vi "XSubMenu-Facade.vi"(0 "Data In":T4, 2 "Display State In":T2={"Items"=[{"Tag"="1", "Name"="1", "Symbol"=0, "Checked"=FALSE, "ParentTag"="t"}], "CellHeight"=0}, 3 "Container State":T3) -> (6 "Data Out":T4, 7 "Display State Out":T2={"Items"=[{"Tag"="1", "Name"="1", "Symbol"=0, "Checked"=FALSE, "ParentTag"="t"}], "CellHeight"=0}, 8 "Action":T1)   [LabVIEW 2020, in "XSubMenu.xctl"]
uses:
  XSubMenu.xctl
  XSubMenu-Data.ctl
  <vilib>/_xctls/Container State.ctl
  XSubMenu-State.ctl
  <vilib>/_xctls/Action.ctl
  <vilib>/_xctls/XControlSupport.lvlib
panel:
  in  "SubMenu":i32(listbox)
  in  "black-ListBg":bool
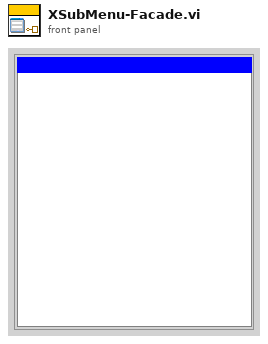
[diagram p1: front panel]
types:
  T1 = typedef "XControlSupport.lvlib/Action.ctl" = cluster{"Data Changed?":bool, "State Changed?":bool, "Action Name":string}
  T2 = typedef "XSubMenu.xctl/XSubMenu-State.ctl" = cluster{"Items":cluster{"Tag":string, "Name":string, "Symbol":i32, "Checked":bool, "ParentTag":string}[], "CellHeight":i32}
  T3 = typedef "XControlSupport.lvlib/Container State.ctl" = cluster{"Indicator?":bool, "Run Mode?":bool, " Refnum":refnum<vi>}
  T4 = typedef "XSubMenu.xctl/XSubMenu-Data.ctl" = i32
  T5 = cluster{"Tag":string, "Name":string, "Symbol":i32, "Checked":bool, "ParentTag":string}[]
  T6 = typedef "imagedata.ctl" = cluster{"image type":i32, "image depth":i32, "image":u8[], "mask":u8[], "colors":u32[], "Rectangle":cluster{"left":i16, "top":i16, "right":i16, "bottom":i16}}
  T7 = typedef "LVPoint32TypeDef.ctl" = cluster{"Horizontal":i32, "Vertical":i32}
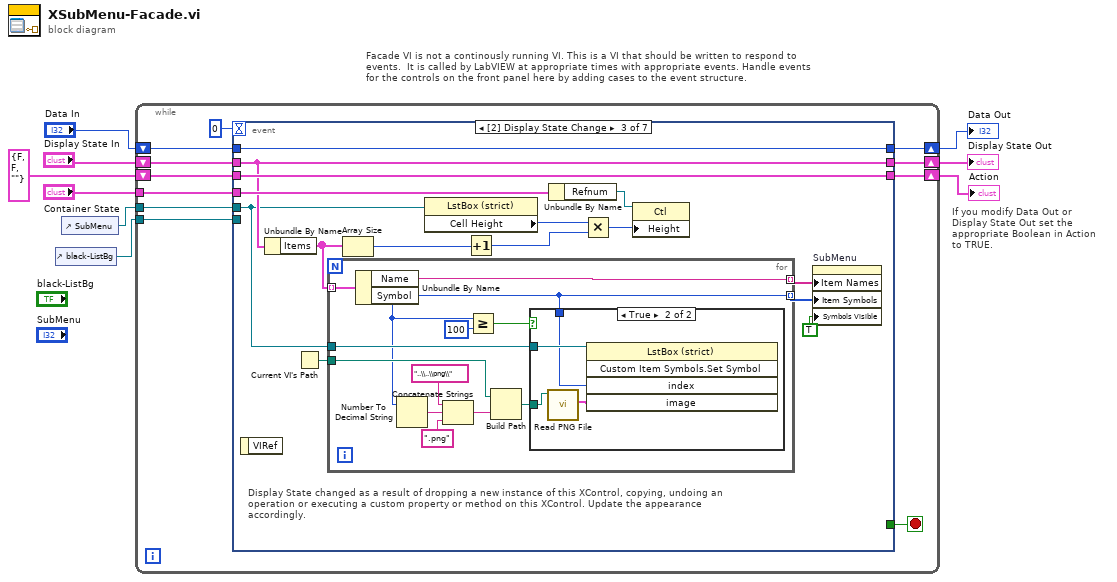
[diagram p0: block diagram]
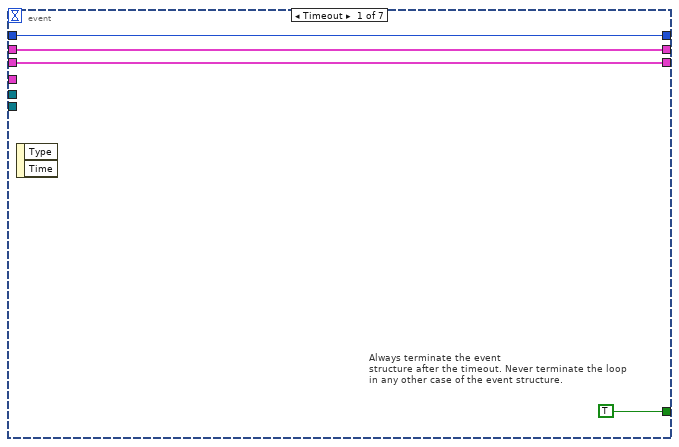
[diagram p2: hidden frame]
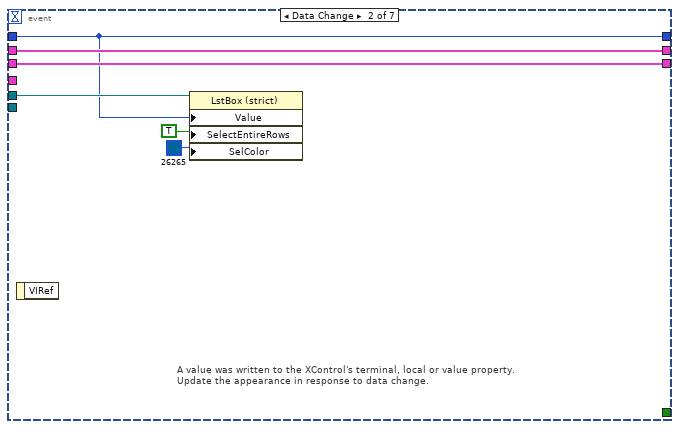
[diagram p3: hidden frame]
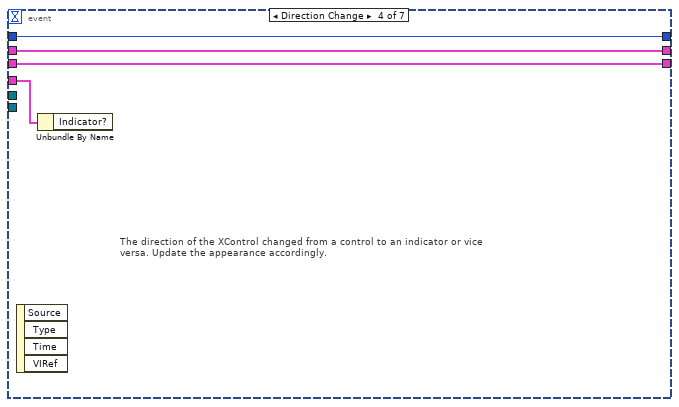
[diagram p5: hidden frame]
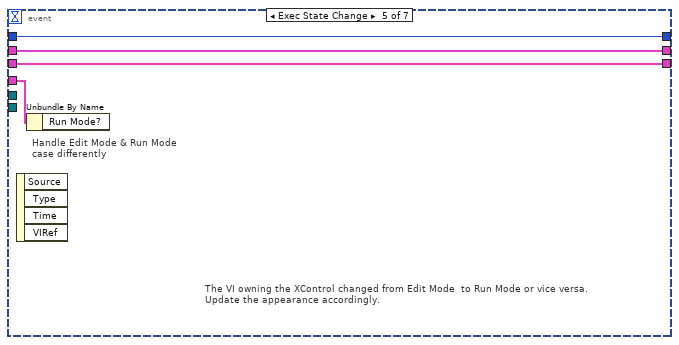
[diagram p6: hidden frame]
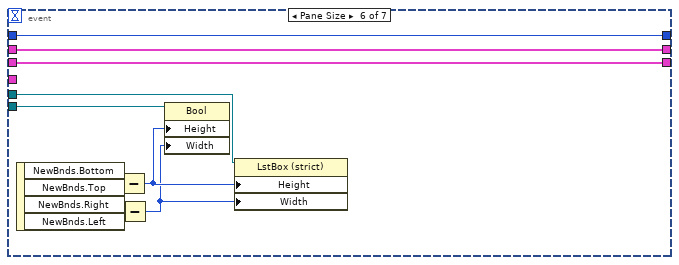
[diagram p7: hidden frame]
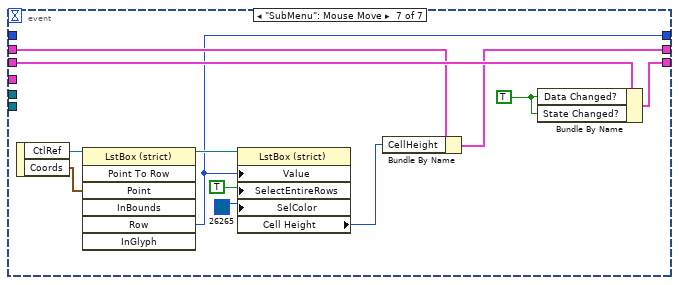
[diagram p8: hidden frame]
diagram:
  # "Facade VI is not a continously running VI. This is a VI that should be written to respond to events.  It is called by LabVIEW at appropriate times with appropriate events. Handle events for the controls on the front panel here by adding cases to the event structure."
  # "If you modify Data Out or\nDisplay State Out set the\nappropriate Boolean in Action\nto TRUE."
  n1 = control-ref of="black-ListBg"() -> (w1:refnum<vi>)
  n2 = control-ref of="SubMenu"() -> (w2:refnum<vi>)
  n3 = while {
    shift-right: [w19] -> w6
    shift-left: "Display State In" -> [w20]
    tunnel: "Container State" -> [w16]
    shift-right: [w14] -> w9
    shift-left: "Data In" -> [w15]
    shift-right: [w12] -> w4
    shift-left: T1 {"Data Changed?"=FALSE, "State Changed?"=FALSE, "Action Name"=""} ("Action") -> [w13]
    tunnel: w2 -> [w11]
    tunnel: w1 -> [w10]
    stop <- w18 stop-if-true
    n4 = event shown="[2] Display State Change" {
      selector: _ -> [_ _ _ _ _ _ _]
      dyn-events: _ -> [_ _ _ _ _ _ _]
      timeout: 0 -> [_ _ _ _ _ _ _]
      tunnel: w20 -> [w22 w29 w35 w64 w68 w71 w84]
      tunnel: [w22 w29 w35 w64 w68 w71 w83] -> w19
      tunnel: [TRUE _ _ _ _ _ _] -> w18
      tunnel: w16 -> [_ _ w36 w65 w69 _ _]
      tunnel: w15 -> [w21 w25 w45 w63 w67 w72 _]
      tunnel: [w21 w25 w45 w63 w67 w72 w81] -> w14
      tunnel: [w23 w30 w44 w62 w66 w70 w86] -> w12
      tunnel: w13 -> [w23 w30 w44 w62 w66 w70 w87]
      tunnel: w11 -> [_ w26 w31 _ _ w76 _]
      tunnel: w10 -> [_ _ _ _ _ w75 _]
      event Timeout {
        # "Always terminate the event\nstructure after the timeout. Never terminate the loop in any other case of the event structure."
        n5 = event-data() -> ()  [unwired: 1 in, 2 out]
      }
      event Data Change {
        # "A value was written to the XControl's terminal, local or value property.\nUpdate the appearance in response to data change."
        n6 = event-data() -> ()  [unwired: 1 in, 1 out]
        n7 = property class="LstBox (strict)"(reference=w26, "Value"=w25, "SelectEntireRows"=TRUE ("Active Row:Cell Font:Bold"), "SelColor"=u32 26265) -> ()  [unwired: 1 in, 2 out]
      }
      event Display State Change {
        # "Display State changed as a result of dropping a new instance of this XControl, copying, undoing an operation or executing a custom property or method on this XControl. Update the appearance accordingly."
        n8 = event-data() -> ()  [unwired: 1 in, 1 out]
        n9 = Unbundle By Name(w35) -> ("Items"=w37:T5)
        n10 = Current VI's Path() -> (path=w32:path)
        n11 = for {
          tunnel: w37 -> [w57] mode=indexing
          tunnel: [w56] -> w43 mode=indexing
          tunnel: [w46] -> w42 mode=indexing
          tunnel: w32 -> [w49]
          tunnel: w31 -> [w48]
          n12 = Unbundle By Name(w57) -> ("Name"=w56:string, "Symbol"=w46:i32)
          n13 = Number To Decimal String(number=w46) -> (decimal integer string=w51:string)  [unwired: 1 in]
          n14 = Concatenate Strings("..\\..\\png\\" ("name or relative path"), w51, ".png" ("string")) -> (w54:string)
          n15 = Greater Or Equal?(x=w46, y=100) -> (x >= y?=w50:bool)
          n16 = Build Path(base path=w49, name or relative path=w54) -> (appended path=w47:path)
          n17 = case shown="True" w50 {
            tunnel: w48 -> [_ w61]
            tunnel: w47 -> [_ w60]
            tunnel: w46 -> [_ w58]
            frame False {
            }
            frame True {
              n18 = call <vilib>:"Read PNG File.vi"("path to PNG file"=w60) -> ("image data"=w59:T6)  [unwired: 8 in, 2 out]
              n19 = invoke class="LstBox (strict)" method="Custom Item Symbols.Set Symbol"(reference=w61, "index"=w58, "image"=w59) -> ()  [unwired: 2 in, 5 out]
            }
          }
        }
        n20 = Array Size(array=w37) -> (size(s)=w34:i32)
        n21 = property class="LstBox (strict)"(reference=w31) -> ("Cell Height"=w39:i32)  [unwired: 1 in, 2 out]
        n22 = Increment(x=w34) -> (x+1=w33:i32)
        n23 = Unbundle By Name(w36) -> ("Refnum"=w40:refnum<vi>)
        n24 = Multiply(x=w39, y=w33) -> (x*y=w38:i32)
        n25 = property class="Ctl"(reference=w40, "Height"=w38) -> ()  [unwired: 1 in, 2 out]
        n26 = property on="SubMenu" class="LstBox (strict)"("Item Names"=w43, "Item Symbols"=w42, "Symbols Visible"=TRUE ("Visible Items:Symbols Visible")) -> ()  [unwired: 2 in, 2 out]
      }
      event Direction Change {
        # "The direction of the XControl changed from a control to an indicator or vice versa. Update the appearance accordingly."
        n27 = event-data() -> ()  [unwired: 1 in, 4 out]
        n28 = Unbundle By Name(w65) -> ()  [unwired: 1 out]
      }
      event Exec State Change {
        # "The VI owning the XControl changed from Edit Mode  to Run Mode or vice versa.\nUpdate the appearance accordingly."
        # "Handle Edit Mode & Run Mode\ncase differently"
        n29 = event-data() -> ()  [unwired: 1 in, 4 out]
        n30 = Unbundle By Name(w69) -> ()  [unwired: 1 out]
      }
      event Pane Size {
        n31 = event-data() -> ("NewBnds.Bottom"=w80:i16, "NewBnds.Top"=w79:i16, "NewBnds.Right"=w78:i16, "NewBnds.Left"=w77:i16)  [unwired: 1 in]
        n32 = Subtract(x=w80, y=w79) -> (x-y=w74:i16)
        n33 = Subtract(x=w78, y=w77) -> (x-y=w73:i16)
        n34 = property class="Bool"(reference=w75, "Height"=w74, "Width"=w73) -> ()  [unwired: 1 in, 2 out]
        n35 = property class="LstBox (strict)"(reference=w76, "Height"=w74, "Width"=w73) -> ()  [unwired: 1 in, 2 out]
      }
      event "SubMenu": Mouse Move {
        w82 = TRUE ("Data Changed?")
        n36 = event-data() -> ("CtlRef"=w91:refnum<vi>, "Coords"=w90:T7)  [unwired: 1 in]
        n37 = invoke class="LstBox (strict)" method="Point To Row"(reference=w91, "Point"=w90) -> (reference out=w89:refnum<vi>, "Row"=w81:i32)  [unwired: 5 in, 5 out]
        n38 = property class="LstBox (strict)"(reference=w89, "Value"=w81, "SelectEntireRows"=TRUE ("Active Row:Cell Font:Bold"), "SelColor"=u32 26265) -> ("Cell Height"=w85:i32)  [unwired: 1 in, 2 out]
        n39 = Bundle By Name(cluster=w84, "CellHeight"=w85) -> (w83:T2)
        n40 = Bundle By Name(cluster=w87, "Data Changed?"=w82, "State Changed?"=w82) -> (w86:T1)
      }
    }
  }
  "Display State Out" <- w6
  "Data Out" <- w9
  "Action" <- w4
